vi "HIL_challenge.vi"() -> ()   [LabVIEW 2019]
panel:
  out "N -> m":string[](array[string])
  in  "file path (use dialog)":path
  out "N":i32[](array[numeric])
  out "m":i32[](array[numeric])
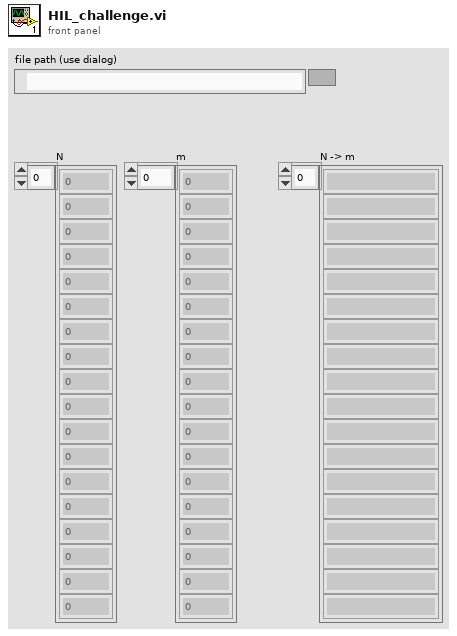
[diagram p1: front panel]
types:
  T1 = enum16{"open", "replace", "create", "open or create", "replace or create", "replace or create with confirmation"}
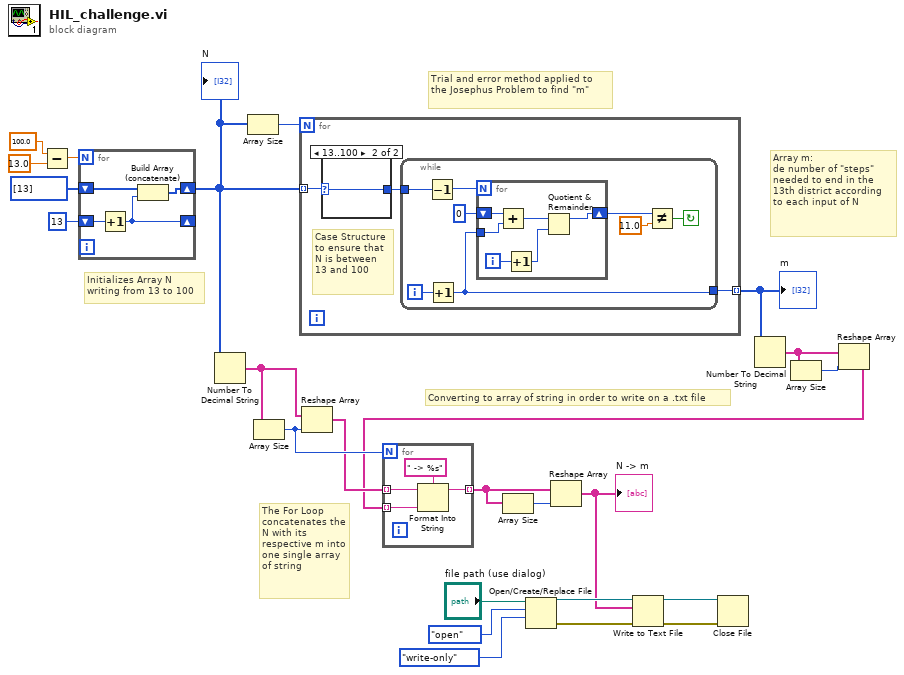
[diagram p0: block diagram]
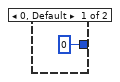
[diagram p2: hidden frame]
diagram:
  # "The For Loop concatenates the N with its respective m into one single array of string"
  # "Converting to array of string in order to write on a .txt file"
  # "Trial and error method applied to the Josephus Problem to find \"m\""
  # "Array m:\nde number of \"steps\" needed to end in the 13th district according to each input of N"
  # "Initializes Array N\nwriting from 13 to 100"
  n1 = Subtract(x=100.0, y=13.0) -> (x-y=w22:dbl)
  n2 = for {
    N: w22 -> [_]
    shift-right: [w28] -> w7
    shift-left: i32[] [13] -> [w27]
    shift-right: [w25] -> _
    shift-left: 13 -> [w26]
    n3 = Increment(x=w26) -> (x+1=w25:i32)
    n4 = Build Array (concatenate)(w27, w25) -> (w28:i32[])
  }
  "N" <- w7
  n5 = Number To Decimal String(number=w7) -> (decimal integer string=w8:string[])  [unwired: 1 in]
  n6 = Array Size(array=w7) -> (size(s)=w19:i32)
  n7 = Array Size(array=w8) -> (size(s)=w6:i32)
  n8 = for {
    N: w19 -> [_]
    tunnel: w7 -> [w30] mode=indexing
    tunnel: [w29] -> w11 mode=indexing
    # "Case Structure to ensure that N is between 13 and 100"
    n9 = case shown="13..100" w30 {
      selector: w30 -> [_ w47]
      tunnel: [0 w47] -> w31
      frame 0, Default {
      }
      frame 13..100 {
      }
    }
    n10 = while {
      tunnel: w31 -> [w33]
      tunnel: [w32] -> w29
      i -> [w35]
      stop <- w38 continue-if-true
      n11 = Decrement(x=w33) -> (x-1=w34:i32)
      n12 = Increment(x=w35) -> (x+1=w32:i32)
      n13 = for {
        N: w34 -> [_]
        shift-right: [w45] -> w36
        shift-left: 0 -> [w42]
        tunnel: w32 -> [w41]
        i -> [w44]
        n14 = Add(x=w42, y=w41) -> (x+y=w40:i32)
        n15 = Increment(x=w44) -> (x+1=w43:i32)
        n16 = Quotient & Remainder(x=w40, y=w43) -> (x-y*floor(x/y)=w45:i32)  [unwired: 1 out]
      }
      n17 = Not Equal?(x=w36, y=11.0) -> (x != y?=w38:bool)
    }
  }
  "m" <- w11
  n18 = Reshape Array(w8, w6) -> (w5:string[])
  n19 = Open/Create/Replace File(file path (use dialog)="file path (use dialog)", operation (0:open)=T1."open", access (0:read/write)=enum16{"read/write", "read-only", "write-only"}."write-only") -> (refnum out=w18:refnum<file>, error out=w17:errorcluster)  [unwired: 3 in, 1 out]
  n20 = Number To Decimal String(number=w11) -> (decimal integer string=w9:string[])  [unwired: 1 in]
  n21 = Array Size(array=w9) -> (size(s)=w10:i32)
  n22 = Reshape Array(w9, w10) -> (w4:string[])
  n23 = for {
    N: w6 -> [_]
    tunnel: w5 -> [w50] mode=indexing
    tunnel: w4 -> [w49] mode=indexing
    tunnel: [w48] -> w2 mode=indexing
    n24 = Format Into String(format string=" -> %s", initial string=w50, w49) -> (resulting string=w48:string)  [unwired: 1 in, 1 out]
  }
  n25 = Array Size(array=w2) -> (size(s)=w3:i32)
  n26 = Reshape Array(w2, w3) -> (w1:string[])
  "N -> m" <- w1
  n27 = Write to Text File(file (use dialog)=w18, text=w1, error in=w17) -> (refnum out=w16:refnum<file>, error out=w15:errorcluster)  [unwired: 1 in, 1 out]
  n28 = Close File(refnum=w16, error in=w15) -> ()  [unwired: 2 out]
